vi "LVFunction_Imop_SlopesCompute_ZonalWavefront.vi"(0 "Phase":refnum<class "Phase.lvclass">, 1 "ComputePhaseSet":refnum<class "ComputePhaseSet.lvclass">, 2 "HasoSlopes":refnum<class "HasoSlopes.lvclass">, 11 "error constant":errorcluster) -> (4 "Phase":refnum<class "Phase.lvclass">, 15 "error out":errorcluster)   [LabVIEW 2020]
doc: "Compute phase from HasoSlopes. Filter some aberrations of reconstructed phase,\ndepending on the filter given in zonal phase reconstruction parameters\nprovided by ComputePhaseSet.\n\n<B>ComputePhaseSetIn</B> : ComputePhaseSet object.\n<B>ComputePhaseSetOut</B> : ComputePhaseSet object.\n<B>HasoSlopes</B> : HasoSlopes object.\n<B>Phase</B> : phase object."
uses:
  ComputePhaseSet.lvclass
  Phase.lvclass
  HasoSlopes.lvclass
  LVClasse_Phase Read SurfaceFloatWithPupil.vi
  LVClass_ComputePhaseSet Read ComputePhaseSet.vi
  LVClass_HasoSlopes Read HasoSlopes _ property.vi
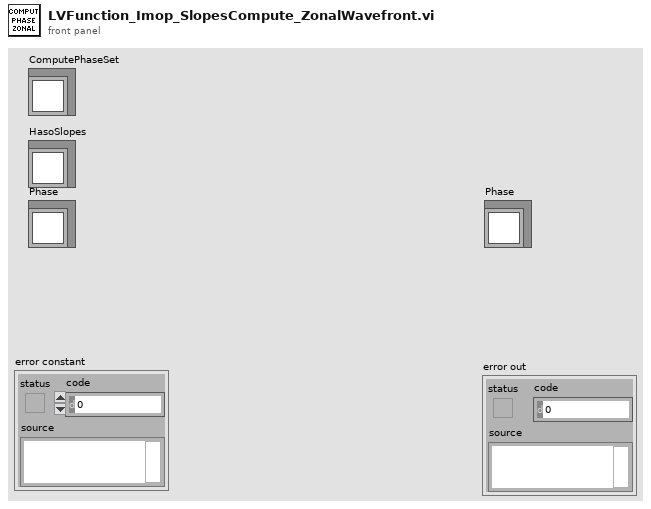
[diagram p1: front panel]
types:
  T1 = typedef "ClassID.ctl" = i64
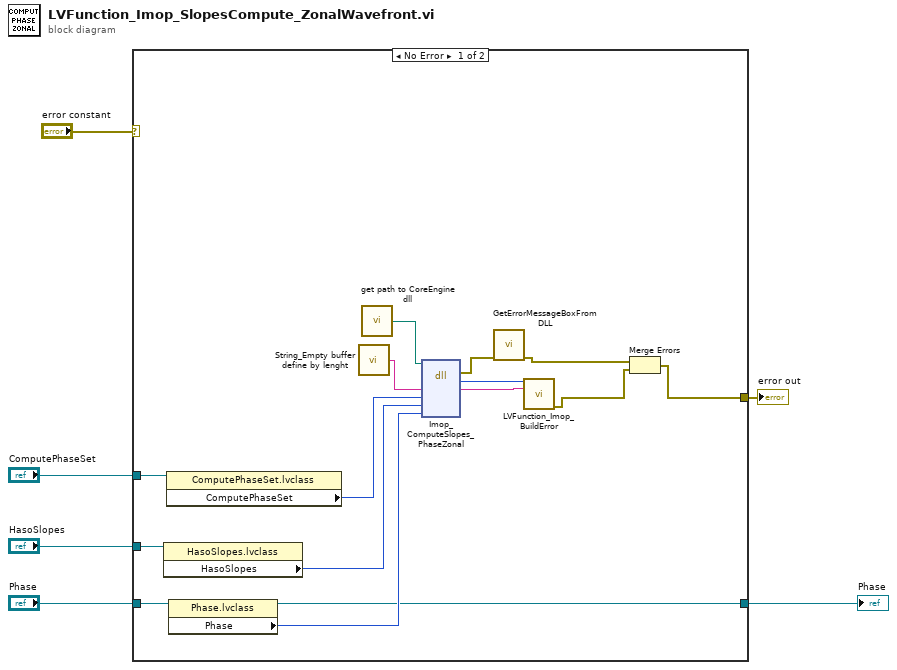
[diagram p0: block diagram]
diagram:
  n1 = case shown="No Error" "error constant" {
    selector: "error constant" -> [_ w23]
    tunnel: "HasoSlopes" -> [w16 _]
    tunnel: "ComputePhaseSet" -> [w15 _]
    tunnel: [w10 w23] -> w4
    tunnel: "Phase" -> [w14 w22]
    tunnel: [w9 w22] -> w2
    frame No Error {
      n2 = property class="HasoSlopes.lvclass"(reference=w16) -> ("HasoSlopes"=w7:T1)  [unwired: 1 in, 2 out]
      n3 = property class="ComputePhaseSet.lvclass"(reference=w15) -> ("ComputePhaseSet"=w8:T1)  [unwired: 1 in, 2 out]
      n4 = property class="Phase.lvclass"(reference=w14) -> (reference out=w9:refnum<class "Phase.lvclass">, "Phase"=w13:T1)  [unwired: 1 in, 1 out]
      n5 = call "String_Empty buffer define by lenght.vi"() -> ("Empty buffer"=w19:string)  [unwired: 1 in]
      n6 = call "get path to CoreEngine dll.vi"() -> ("path to wavekit library"=w18:path)  [unwired: 14 in, 1 out]
      n7 = dll-call lib="D:/FLE/0.Code/CoreEngine4_Suite/LV2011_interface/DLLs/c_interface_vc100.dll" fn="Imop_ComputeSlopes_PhaseZonal"(path in=w18, "message"=w19, "ComputePhaseSet"=w8, "HasoSlopes"=w7, "Phase"=w13) -> (error out=w17:errorcluster, "return type"=w21:i32, "message"=w20:string)  [unwired: 5 in, 1 out]
      n8 = call "GetErrorMessageBoxFromDLL.vi"("error IN"=w17) -> ("error OUT"=w12:errorcluster)  [unwired: 10 in]
      n9 = call "LVFunction_Imop_BuildError.vi"("code"=w21, "String to Prepend to source (\"\")"=w20) -> ("error out"=w11:errorcluster)  [unwired: 13 in]
      n10 = Merge Errors(w12, w11) -> (w10:errorcluster)
    }
    frame Error {
    }
  }
  "error out" <- w4
  "Phase" <- w2
